vi "分层图显示1.1.1（刻度色码）.vi"(11 "IN":string) -> (3 "OUT":string)   [LabVIEW 2016]
uses:
  <vilib>/Utility/file.llb/Read Delimited Spreadsheet (DBL).vi
panel:
  in  "色码":u32[](array[colorbox])=[16726058, 16774930, 0]
  out "导入进度":u8(slide) scale=0.0..100.0
  in  "min":dbl format="%#_4e"
  in  "max":dbl format="%#_4e"
  in  "ESC":bool
  out "分层图":dbl[][](graph)
  in  "NEXT":bool
  in  "层数:":i32
  out "数组":dbl[][][](array[numeric])
  # "强度表"
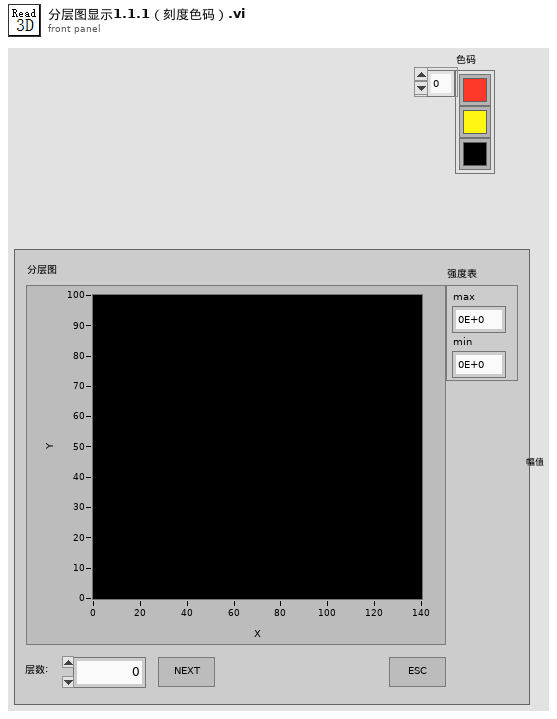
[diagram p1: front panel]
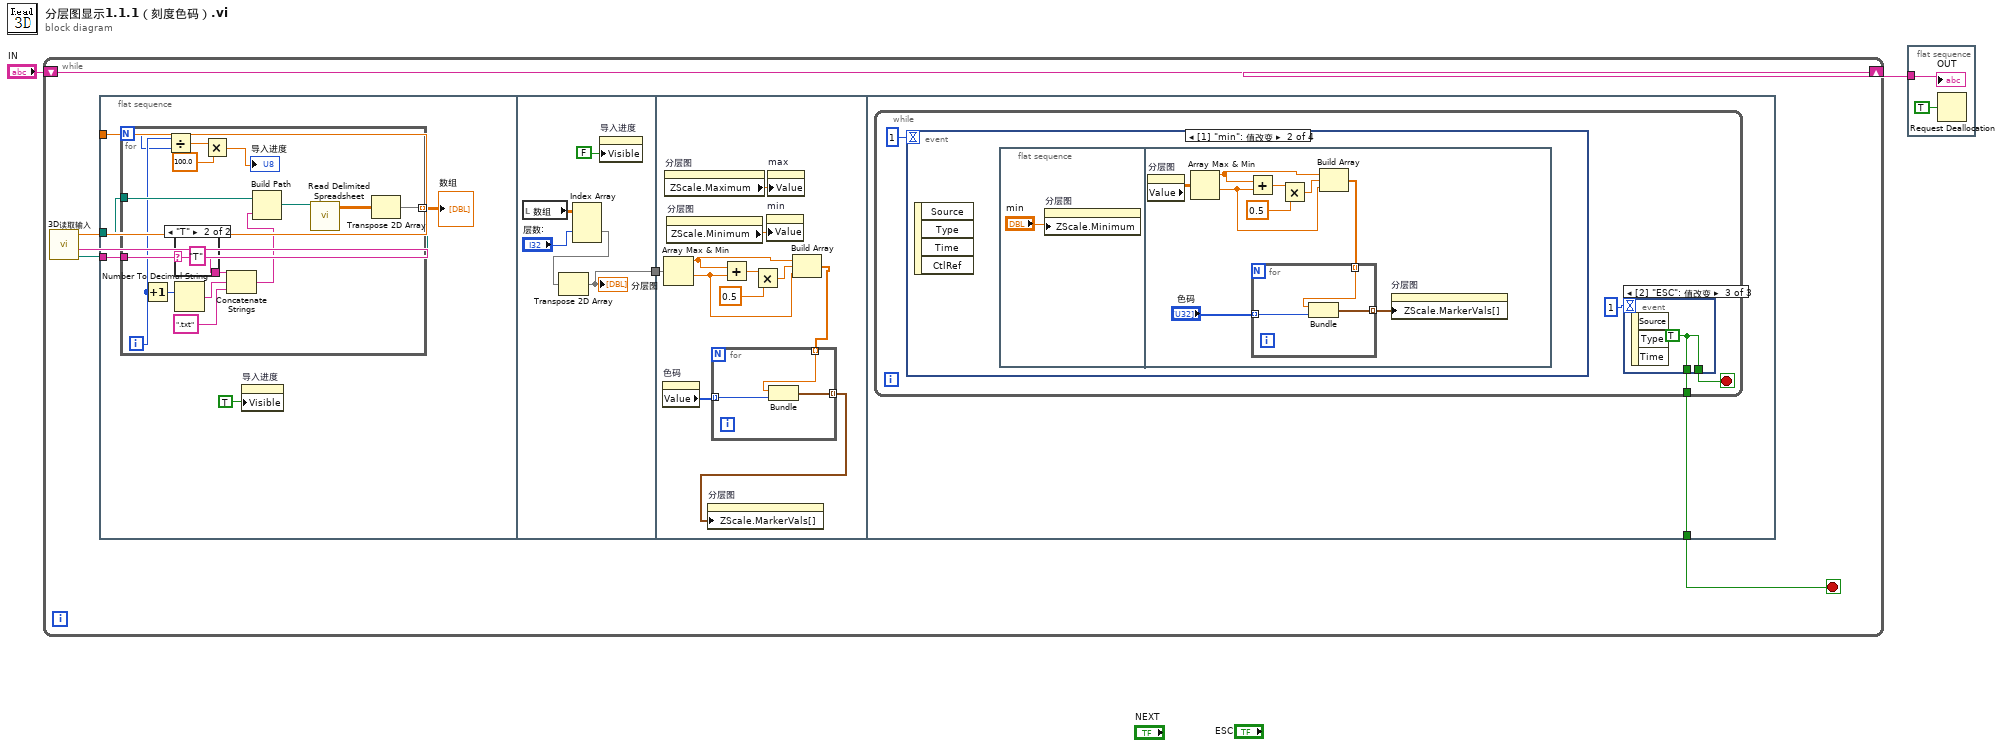
[diagram p0: block diagram]
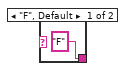
[diagram p2: hidden frame]
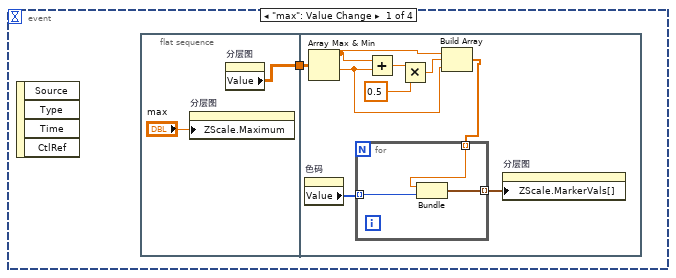
[diagram p3: hidden frame]
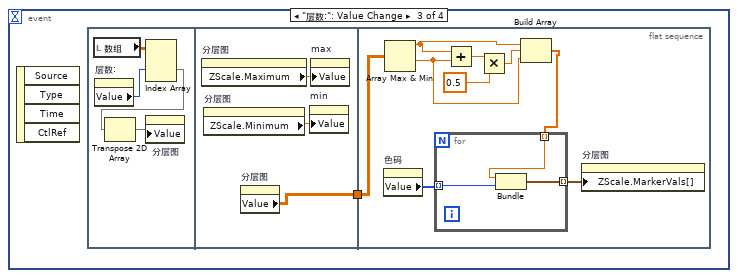
[diagram p4: hidden frame]
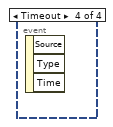
[diagram p5: hidden frame]
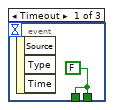
[diagram p6: hidden frame]
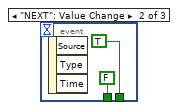
[diagram p7: hidden frame]
diagram:
  n1 = while {
    shift-right: [w8] -> w1
    shift-left: "IN" -> [w8]
    stop <- w7 stop-if-true
    n2 = call "3D读取输入.vi"() -> ("文件读取路径"=w4:path, "时域谱or频域谱"=w5:string, "行总数"=w6:dbl)  [unwired: 9 in]
    n3 = flat-sequence {
      tunnel: w6 -> [w12]
      tunnel: w5 -> [w11]
      tunnel: w4 -> [w10]
      tunnel: [w31] -> w3
      tunnel: w3 -> [w36]
      tunnel: [w50] -> w7
      frame #0 {
        n4 = for {
          N: w12 -> [w17]
          tunnel: [w27] -> w13 mode=indexing
          tunnel: w11 -> [w20]
          tunnel: w10 -> [w19]
          i -> [w18]
          n5 = Increment(x=w18) -> (x+1=w23:i32)
          n6 = Divide(x=w18, y=w17) -> (x/y=w16:dbl)
          n7 = case shown="\"T\"" w20 {
            tunnel: ["F" "T"] -> w25
            frame "F", Default {
            }
            frame "T" {
            }
          }
          n8 = Number To Decimal String(number=w23) -> (decimal integer string=w22:string)  [unwired: 1 in]
          n9 = Multiply(x=w16, y=100.0) -> (x*y=→"导入进度":dbl)
          n10 = Concatenate Strings(w25, w22, ".txt") -> (w24:string)
          n11 = Build Path(base path=w19, name or relative path=w24) -> (appended path=w26:path)
          n12 = call-poly <vilib>:"Read Delimited Spreadsheet.vi"("file path (dialog if empty)"=w26) -> ("all rows"=w28:dbl[][])  [unwired: 9 in, 5 out]
          n13 = Transpose 2D Array(2D array=w28) -> (transposed array=w27:dbl[][])
        }
        "数组" <- w13
        n14 = property on="导入进度" class="Slide (严格)"("Visible"=TRUE ("可见")) -> ()  [unwired: 2 in, 2 out]
      }
      frame #1 {
        n15 = local read "数组"() -> (w34:dbl[][][])
        n16 = Index Array(array=w34, index (dim 1)="层数:") -> (element=w32:dbl[][])  [unwired: 2 in]
        n17 = Transpose 2D Array(2D array=w32) -> (transposed array=w31:dbl[][])
        "分层图" <- w31
        n18 = property on="导入进度" class="Slide (严格)"("Visible"=FALSE ("可见")) -> ()  [unwired: 2 in, 2 out]
      }
      frame #2 {
        n19 = property on="色码" class="Arr (严格)"() -> ("Value"=w43:u32[])  [unwired: 2 in, 2 out]
        n20 = Array Max & Min(array=w36) -> (max value=w39:dbl, min value=w41:dbl)  [unwired: 2 out]
        n21 = property on="分层图" class="IntGraph (严格)"() -> ("ZScale.Maximum"=w45:dbl)  [unwired: 2 in, 2 out]
        n22 = property on="分层图" class="IntGraph (严格)"() -> ("ZScale.Minimum"=w46:dbl)  [unwired: 2 in, 2 out]
        n23 = Add(x=w39, y=w41) -> (x+y=w37:dbl)
        n24 = Multiply(x=w37, y=0.5) -> (x*y=w40:dbl)
        n25 = property on="min" class="DigNum (严格)"("Value"=w46) -> ()  [unwired: 2 in, 2 out]
        n26 = property on="max" class="DigNum (严格)"("Value"=w45) -> ()  [unwired: 2 in, 2 out]
        n27 = Build Array(w39, w40, w41) -> (w44:dbl[])
        n28 = for {
          tunnel: w44 -> [w49] mode=indexing
          tunnel: w43 -> [w48] mode=indexing
          tunnel: [w47] -> w42 mode=indexing
          n29 = Bundle(w49, "颜色盒"=w48) -> (w47:cluster{dbl, "颜色盒":u32})  [unwired: 1 in]
        }
        n30 = property on="分层图" class="IntGraph (严格)"("ZScale.MarkerVals[]"=w42) -> ()  [unwired: 2 in, 2 out]
      }
      frame #3 {
        n31 = while {
          tunnel: [w53] -> w50
          stop <- w54 stop-if-true
          n32 = event shown="[1] \"min\": 值改变" {
            selector: _ -> [_ _ _ _]
            dyn-events: _ -> [_ _ _ _]
            timeout: 1 -> [_ _ _ _]
            event "max": Value Change {
              n33 = event-data() -> ()  [unwired: 1 in, 4 out]
              n34 = flat-sequence {
                tunnel: [w56] -> w55
                tunnel: w55 -> [w58]
                frame #0 {
                  n35 = property on="分层图" class="IntGraph (严格)"("ZScale.Maximum"="max") -> ()  [unwired: 2 in, 2 out]
                  n36 = property on="分层图" class="IntGraph (严格)"() -> ("Value"=w56:dbl[][])  [unwired: 2 in, 2 out]
                }
                frame #1 {
                  n37 = property on="色码" class="Arr (严格)"() -> ("Value"=w65:u32[])  [unwired: 2 in, 2 out]
                  n38 = Array Max & Min(array=w58) -> (max value=w61:dbl, min value=w63:dbl)  [unwired: 2 out]
                  n39 = Add(x=w61, y=w63) -> (x+y=w59:dbl)
                  n40 = Multiply(x=w59, y=0.5) -> (x*y=w62:dbl)
                  n41 = Build Array(w61, w62, w63) -> (w66:dbl[])
                  n42 = for {
                    tunnel: w66 -> [w69] mode=indexing
                    tunnel: w65 -> [w68] mode=indexing
                    tunnel: [w67] -> w64 mode=indexing
                    n43 = Bundle(w69, "颜色盒"=w68) -> (w67:cluster{dbl, "颜色盒":u32})  [unwired: 1 in]
                  }
                  n44 = property on="分层图" class="IntGraph (严格)"("ZScale.MarkerVals[]"=w64) -> ()  [unwired: 2 in, 2 out]
                }
              }
            }
            event "min": Value Change {
              n45 = event-data() -> ()  [unwired: 1 in, 4 out]
              n46 = flat-sequence {
                frame #0 {
                  n47 = property on="分层图" class="IntGraph (严格)"("ZScale.Minimum"="min") -> ()  [unwired: 2 in, 2 out]
                }
                frame #1 {
                  n48 = property on="分层图" class="IntGraph (严格)"() -> ("Value"=w72:dbl[][])  [unwired: 2 in, 2 out]
                  n49 = Array Max & Min(array=w72) -> (max value=w75:dbl, min value=w77:dbl)  [unwired: 2 out]
                  n50 = Add(x=w75, y=w77) -> (x+y=w73:dbl)
                  n51 = Multiply(x=w73, y=0.5) -> (x*y=w76:dbl)
                  n52 = Build Array(w75, w76, w77) -> (w78:dbl[])
                  n53 = for {
                    tunnel: w78 -> [w82] mode=indexing
                    tunnel: "色码" -> [w81] mode=indexing
                    tunnel: [w80] -> w79 mode=indexing
                    n54 = Bundle(w82, "颜色盒"=w81) -> (w80:cluster{dbl, "颜色盒":u32})  [unwired: 1 in]
                  }
                  n55 = property on="分层图" class="IntGraph (严格)"("ZScale.MarkerVals[]"=w79) -> ()  [unwired: 2 in, 2 out]
                }
              }
            }
            event "层数:": Value Change {
              n56 = event-data() -> ()  [unwired: 1 in, 4 out]
              n57 = flat-sequence {
                tunnel: [w88] -> w83
                tunnel: w83 -> [w91]
                frame #0 {
                  n58 = local read "数组"() -> (w86:dbl[][][])
                  n59 = property on="层数:" class="DigNum (严格)"() -> ("Value"=w87:i32)  [unwired: 2 in, 2 out]
                  n60 = Index Array(array=w86, index (dim 1)=w87) -> (element=w85:dbl[][])  [unwired: 2 in]
                  n61 = Transpose 2D Array(2D array=w85) -> (transposed array=w84:dbl[][])
                  n62 = property on="分层图" class="IntGraph (严格)"("Value"=w84) -> ()  [unwired: 2 in, 2 out]
                }
                frame #1 {
                  n63 = property on="分层图" class="IntGraph (严格)"() -> ("ZScale.Maximum"=w90:dbl)  [unwired: 2 in, 2 out]
                  n64 = property on="分层图" class="IntGraph (严格)"() -> ("ZScale.Minimum"=w89:dbl)  [unwired: 2 in, 2 out]
                  n65 = property on="分层图" class="IntGraph (严格)"() -> ("Value"=w88:dbl[][])  [unwired: 2 in, 2 out]
                  n66 = property on="min" class="DigNum (严格)"("Value"=w89) -> ()  [unwired: 2 in, 2 out]
                  n67 = property on="max" class="DigNum (严格)"("Value"=w90) -> ()  [unwired: 2 in, 2 out]
                }
                frame #2 {
                  n68 = property on="色码" class="Arr (严格)"() -> ("Value"=w98:u32[])  [unwired: 2 in, 2 out]
                  n69 = Array Max & Min(array=w91) -> (max value=w94:dbl, min value=w96:dbl)  [unwired: 2 out]
                  n70 = Add(x=w94, y=w96) -> (x+y=w92:dbl)
                  n71 = Multiply(x=w92, y=0.5) -> (x*y=w95:dbl)
                  n72 = Build Array(w94, w95, w96) -> (w99:dbl[])
                  n73 = for {
                    tunnel: w99 -> [w102] mode=indexing
                    tunnel: w98 -> [w101] mode=indexing
                    tunnel: [w100] -> w97 mode=indexing
                    n74 = Bundle(w102, "颜色盒"=w101) -> (w100:cluster{dbl, "颜色盒":u32})  [unwired: 1 in]
                  }
                  n75 = property on="分层图" class="IntGraph (严格)"("ZScale.MarkerVals[]"=w97) -> ()  [unwired: 2 in, 2 out]
                }
              }
            }
            event Timeout {
              n76 = event-data() -> ()  [unwired: 1 in, 3 out]
            }
          }
          n77 = event shown="[2] \"ESC\": 值改变" {
            selector: _ -> [_ _ _]
            dyn-events: _ -> [_ _ _]
            timeout: 1 -> [_ _ _]
            tunnel: [w103 TRUE w106] -> w54
            tunnel: [w103 FALSE w106] -> w53
            event Timeout {
              w103 = FALSE
              n78 = event-data() -> ()  [unwired: 1 in, 3 out]
            }
            event "NEXT": Value Change {
              n79 = event-data() -> ()  [unwired: 1 in, 3 out]
            }
            event "ESC": Value Change {
              w106 = TRUE
              n80 = event-data() -> ()  [unwired: 1 in, 3 out]
            }
          }
        }
      }
    }
  }
  n81 = flat-sequence {
    tunnel: w1 -> [w108]
    frame #0 {
      n82 = Request Deallocation(TRUE ("标志")) -> ()
      "OUT" <- w108
    }
  }
